vi "svx_DAQ_UpdateTriggerSection.vi"(5 "State":T1={"Channel Info Array"=[], "Timing Mode"=enum."Time", "Timing Control 1"=25600.0, "Timing Control 2"=2560.0, "Timing Control 3"=16, "Timing Indicator 1"=0.1, "Reference Visible?"=FALSE, "Reference Type"=enum."<none>", "Tachometer Channel"="", "Tach Pulses Per Rev"=1, "Tach Direction"=enum."CW", "Tach Slope"=enum."Rising", "Tach Threshold"=0.0, "Trigger Channel"="", "Trigger Level"=20.0, "Pretrigger Samples"=1, "Trigger Slope"=enum."Falling", "Trigger Hysteresis"=0.0, "Logging Visible?"=FALSE, "Enable Logging"=FALSE, "Logfile Path"=path "c:/test.tdms"} {"Timing Control 2" format="%#_6f"; "Channel Info Array"."Max" min=0.0 format="± %^#_4g"; "Channel Info Array"."Channel Type" items=["Voltage (V)"=0, "Charge (C)"=9, "-"=99, "SPL (Pa)"=3, "Force (lbf)"=6, "Force (N)"=1, "Acceleration (g) - IEPE"=2, "Acceleration (g) - Charge"=12, "Acceleration (g) - 4 wire DC Voltage"=22, "Velocity (in/s)"=7, "Velocity (mm/s)"=8, "Prox Probe (mil)"=4, "Prox Probe (mm)"=5]}, 9 "Reference Cluster":T11, 11 "error in (no error)":errorcluster) -> (6 "State Out":T1={"Channel Info Array"=[], "Timing Mode"=enum."Time", "Timing Control 1"=25600.0, "Timing Control 2"=2560.0, "Timing Control 3"=16, "Timing Indicator 1"=0.1, "Reference Visible?"=FALSE, "Reference Type"=enum."<none>", "Tachometer Channel"="", "Tach Pulses Per Rev"=1, "Tach Direction"=enum."CW", "Tach Slope"=enum."Rising", "Tach Threshold"=0.0, "Trigger Channel"="", "Trigger Level"=20.0, "Pretrigger Samples"=1, "Trigger Slope"=enum."Falling", "Trigger Hysteresis"=0.0, "Logging Visible?"=FALSE, "Enable Logging"=FALSE, "Logfile Path"=path "c:/test.tdms"} caption="State" {"Timing Control 2" format="%#_6f"; "Channel Info Array"."Max" min=0.0 format="± %^#_4g"; "Channel Info Array"."Channel Type" items=["Voltage (V)"=0, "Charge (C)"=9, "-"=99, "SPL (Pa)"=3, "Force (lbf)"=6, "Force (N)"=1, "Acceleration (g) - IEPE"=2, "Acceleration (g) - Charge"=12, "Acceleration (g) - 4 wire DC Voltage"=22, "Velocity (in/s)"=7, "Velocity (mm/s)"=8, "Prox Probe (mil)"=4, "Prox Probe (mm)"=5]}, 10 "Reference Cluster Out":T11, 15 "error out":errorcluster)   [LabVIEW 2017, in "SVX NI-DAQmx AI Configuration XControl.xctl"]
uses:
  <vilib>/addons/Sound and Vibration/svt_DAQmx/Configuration XControl/SVX NI-DAQmx AI Configuration XControl.xctl
  <vilib>/addons/Sound and Vibration/svt_DAQmx/Configuration XControl/SubVIs/svx_DAQ_State.ctl
  <vilib>/addons/Sound and Vibration/svt_DAQmx/Configuration XControl/Controls/svx_DAQ_ChannelInfo.ctl
  <vilib>/addons/Sound and Vibration/svt_DAQmx/Configuration XControl/Controls/svx_DAQ_ChannelType.ctl
  <vilib>/addons/Sound and Vibration/svt_DAQmx/Configuration XControl/Controls/svx_DAQ_Coupling.ctl
  <vilib>/addons/Sound and Vibration/svt_DAQmx/Configuration XControl/Controls/svx_DAQ_Excitation.ctl
  <vilib>/addons/Sound and Vibration/svt_DAQmx/Configuration XControl/Controls/svx_DAQ_TimingType.ctl
  <vilib>/addons/Sound and Vibration/svt_DAQmx/Configuration XControl/Controls/svx_DAQ_ReferenceType.ctl
  <vilib>/addons/Sound and Vibration/svt_DAQmx/Configuration XControl/Controls/svx_DAQ_RotationDirection.ctl
  <vilib>/addons/Sound and Vibration/svt_DAQmx/Configuration XControl/Controls/svx_DAQ_Tach_Slope.ctl
  <vilib>/addons/Sound and Vibration/svt_DAQmx/Configuration XControl/Controls/svx_DAQ_Trigger_Slope.ctl
  <vilib>/addons/Sound and Vibration/svt_DAQmx/Configuration XControl/Controls/svx_DAQ_ControlRefs.ctl
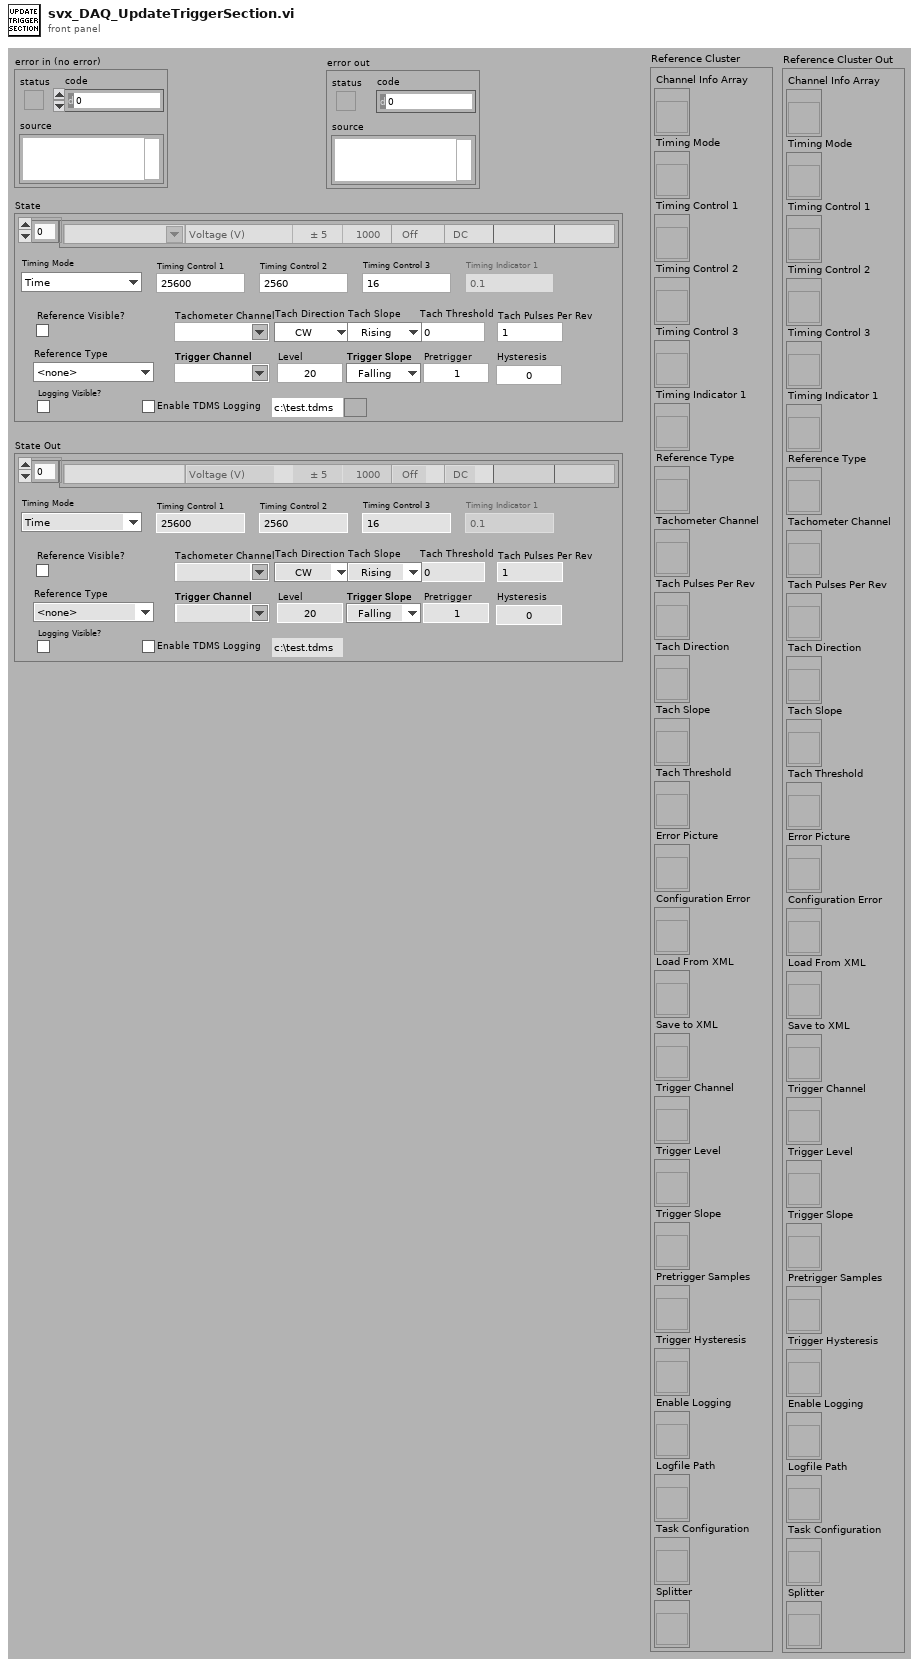
[diagram p1: front panel]
types:
  T1 = typedef "SVX NI-DAQmx AI Configuration XControl.xctl/svx_DAQ_State.ctl" = cluster{"Channel Info Array":T2[], "Timing Mode":T6, "Timing Control 1":dbl, "Timing Control 2":dbl, "Timing Control 3":i32, "Timing Indicator 1":dbl, "Reference Visible?":bool, "Reference Type":T7, "Tachometer Channel":string, "Tach Pulses Per Rev":i32, "Tach Direction":T8, "Tach Slope":T9, "Tach Threshold":dbl, "Trigger Channel":string, "Trigger Level":dbl, "Pretrigger Samples":i32, "Trigger Slope":T10, "Trigger Hysteresis":dbl, "Logging Visible?":bool, "Enable Logging":bool, "Logfile Path":path}
  T2 = typedef "SVX NI-DAQmx AI Configuration XControl.xctl/svx_DAQ_ChannelInfo.ctl" = cluster{"Initialized?":bool, "DAQmx Channel":tag, "Channel Type":T3, "Max":dbl, "Sensitivity":dbl, "Excitation":bool, "Coupling":T4, "Location":string, "Orientation":string, "excitation":T5}
  T3 = typedef "SVX NI-DAQmx AI Configuration XControl.xctl/svx_DAQ_ChannelType.ctl" = u16
  T4 = typedef "SVX NI-DAQmx AI Configuration XControl.xctl/svx_DAQ_Coupling.ctl" = enum16{"AC", "DC"}
  T5 = typedef "svx_DAQ_Excitation.ctl" = enum16{"Off", "Min", "Max"}
  T6 = typedef "SVX NI-DAQmx AI Configuration XControl.xctl/svx_DAQ_TimingType.ctl" = enum16{"Time", "Frequency", "Order"}
  T7 = typedef "SVX NI-DAQmx AI Configuration XControl.xctl/svx_DAQ_ReferenceType.ctl" = enum16{"<none>", "Analog Tachometer", "Analog SW Trigger"}
  T8 = typedef "SVX NI-DAQmx AI Configuration XControl.xctl/svx_DAQ_RotationDirection.ctl" = enum16{"CW", "CCW"}
  T9 = typedef "SVX NI-DAQmx AI Configuration XControl.xctl/svx_DAQ_Tach_Slope.ctl" = enum16{"Rising", "Falling"}
  T10 = typedef "SVX NI-DAQmx AI Configuration XControl.xctl/svx_DAQ_Trigger_Slope.ctl" = enum16{"Falling", "Rising"}
  T11 = typedef "SVX NI-DAQmx AI Configuration XControl.xctl/svx_DAQ_ControlRefs.ctl" = cluster{"Channel Info Array":refnum<vi>, "Timing Mode":refnum<vi>, "Timing Control 1":refnum<vi>, "Timing Control 2":refnum<vi>, "Timing Control 3":refnum<vi>, "Timing Indicator 1":refnum<vi>, "Reference Type":refnum<vi>, "Tachometer Channel":refnum<vi>, "Tach Pulses Per Rev":refnum<vi>, "Tach Direction":refnum<vi>, "Tach Slope":refnum<vi>, "Tach Threshold":refnum<vi>, "Error Picture":refnum<vi>, "Configuration Error":refnum<vi>, "Load From XML":refnum<vi>, "Save to XML":refnum<vi>, "Trigger Channel":refnum<vi>, "Trigger Level":refnum<vi>, "Trigger Slope":refnum<vi>, "Pretrigger Samples":refnum<vi>, "Trigger Hysteresis":refnum<vi>, "Enable Logging":refnum<vi>, "Logfile Path":refnum<vi>, "Task Configuration":refnum<vi>, "Splitter":refnum<vi>}
  T12 = enum8{"Enabled", "Disabled", "Disabled and Grayed Out"}
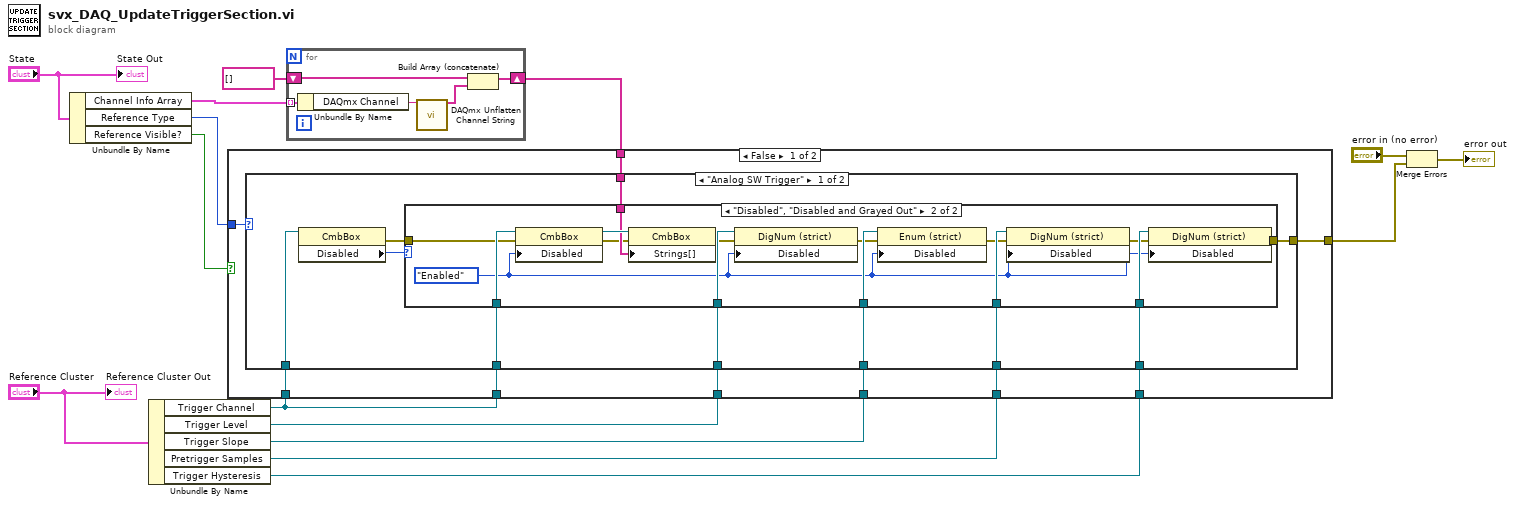
[diagram p0: block diagram]
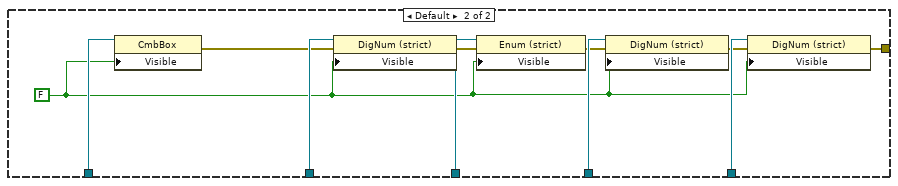
[diagram p3: hidden frame]
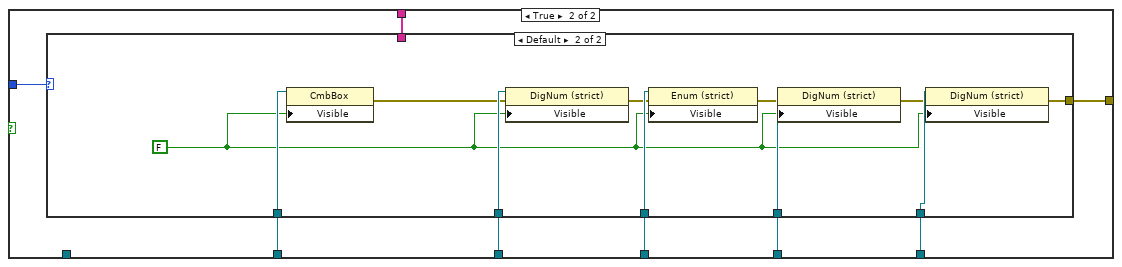
[diagram p4: hidden frame]
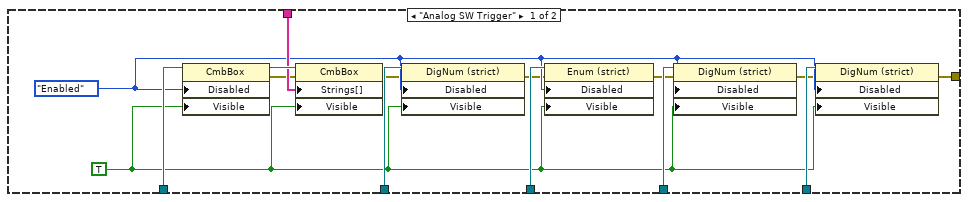
[diagram p5: hidden frame]
diagram:
  n1 = Unbundle By Name("State") -> ("Channel Info Array"=w11:T2[], "Reference Type"=w6:T7, "Reference Visible?"=w2:bool)
  n2 = Unbundle By Name("Reference Cluster") -> ("Trigger Channel"=w1:refnum<vi>, "Trigger Level"=w14:refnum<vi>, "Trigger Slope"=w15:refnum<vi>, "Pretrigger Samples"=w13:refnum<vi>, "Trigger Hysteresis"=w12:refnum<vi>)
  n3 = for {
    tunnel: w11 -> [w20] mode=indexing
    shift-right: [w17] -> w9
    shift-left: string[] [] ("Strings []") -> [w18]
    n4 = Unbundle By Name(w20) -> ("DAQmx Channel"=w19:tag)
    n5 = call <vilib>:"DAQmx Unflatten Channel String.vi"("names in"=w19) -> ("names out"=w16:string[])  [unwired: 13 in, 1 out]
    n6 = Build Array (concatenate)(w18, w16) -> (w17:string[])
  }
  n7 = case shown="False" w2 {
    tunnel: w15 -> [w24 w74]
    tunnel: w14 -> [w25 w73]
    tunnel: w13 -> [w23 w72]
    tunnel: w12 -> [w22 w71]
    tunnel: w9 -> [w27 w70]
    tunnel: [w29 w69] -> w8
    tunnel: w6 -> [w28 w68]
    tunnel: w1 -> [w26 w67]
    tunnel: w1 -> [w21 _]
    frame False {
      n8 = case shown="\"Analog SW Trigger\"" w28 {
        tunnel: w24 -> [w39 w66]
        tunnel: w25 -> [w38 w65]
        tunnel: w26 -> [w37 w64]
        tunnel: w23 -> [w36 w63]
        tunnel: w22 -> [w35 w62]
        tunnel: w27 -> [w34 _]
        tunnel: [w33 w58] -> w29
        tunnel: w21 -> [w32 _]
        frame "Analog SW Trigger" {
          n9 = property class="CmbBox"(reference=w32) -> (error out=w30:errorcluster, "Disabled"=w31:T12)  [unwired: 1 in, 1 out]
          n10 = case shown="\"Disabled\", \"Disabled and Grayed Out\"" w31 {
            tunnel: w39 -> [_ w55]
            tunnel: w38 -> [_ w54]
            tunnel: w37 -> [_ w53]
            tunnel: w36 -> [_ w52]
            tunnel: w35 -> [_ w51]
            tunnel: w34 -> [_ w49]
            tunnel: [w40 w43] -> w33
            tunnel: w30 -> [w40 w41]
            frame "Enabled", Default {
            }
            frame "Disabled", "Disabled and Grayed Out" {
              w42 = T12."Enabled" ("Disabled")
              n11 = property class="CmbBox"(reference=w53, error in=w41, "Disabled"=w42) -> (reference out=w50:refnum<vi>, error out=w48:errorcluster)
              n12 = property class="CmbBox"(reference=w50, error in=w48, "Strings[]"=w49) -> (error out=w47:errorcluster)  [unwired: 1 out]
              n13 = property class="DigNum (strict)"(reference=w54, error in=w47, "Disabled"=w42) -> (error out=w46:errorcluster)  [unwired: 1 out]
              n14 = property class="Enum (strict)"(reference=w55, error in=w46, "Disabled"=w42) -> (error out=w45:errorcluster)  [unwired: 1 out]
              n15 = property class="DigNum (strict)"(reference=w52, error in=w45, "Disabled"=w42) -> (error out=w44:errorcluster)  [unwired: 1 out]
              n16 = property class="DigNum (strict)"(reference=w51, error in=w44, "Disabled"=w42) -> (error out=w43:errorcluster)  [unwired: 1 out]
            }
          }
        }
        frame Default {
          w56 = FALSE ("Visible")
          n17 = property class="CmbBox"(reference=w64, "Visible"=w56) -> (error out=w57:errorcluster)  [unwired: 1 in, 1 out]
          n18 = property class="DigNum (strict)"(reference=w65, error in=w57, "Visible"=w56) -> (error out=w61:errorcluster)  [unwired: 1 out]
          n19 = property class="Enum (strict)"(reference=w66, error in=w61, "Visible"=w56) -> (error out=w60:errorcluster)  [unwired: 1 out]
          n20 = property class="DigNum (strict)"(reference=w63, error in=w60, "Visible"=w56) -> (error out=w59:errorcluster)  [unwired: 1 out]
          n21 = property class="DigNum (strict)"(reference=w62, error in=w59, "Visible"=w56) -> (error out=w58:errorcluster)  [unwired: 1 out]
        }
      }
    }
    frame True {
      n22 = case shown="Default" w68 {
        tunnel: w74 -> [w89 w100]
        tunnel: w73 -> [w88 w99]
        tunnel: w67 -> [w87 w98]
        tunnel: w72 -> [w86 w97]
        tunnel: w71 -> [w85 w96]
        tunnel: w70 -> [w83 _]
        tunnel: [w76 w92] -> w69
        frame "Analog SW Trigger" {
          w75 = TRUE ("Visible")
          w82 = T12."Enabled" ("Disabled")
          n23 = property class="CmbBox"(reference=w87, "Disabled"=w82, "Visible"=w75) -> (reference out=w84:refnum<vi>, error out=w81:errorcluster)  [unwired: 1 in]
          n24 = property class="CmbBox"(reference=w84, error in=w81, "Strings[]"=w83, "Visible"=w75) -> (error out=w80:errorcluster)  [unwired: 1 out]
          n25 = property class="DigNum (strict)"(reference=w88, error in=w80, "Disabled"=w82, "Visible"=w75) -> (error out=w79:errorcluster)  [unwired: 1 out]
          n26 = property class="Enum (strict)"(reference=w89, error in=w79, "Disabled"=w82, "Visible"=w75) -> (error out=w78:errorcluster)  [unwired: 1 out]
          n27 = property class="DigNum (strict)"(reference=w86, error in=w78, "Disabled"=w82, "Visible"=w75) -> (error out=w77:errorcluster)  [unwired: 1 out]
          n28 = property class="DigNum (strict)"(reference=w85, error in=w77, "Disabled"=w82, "Visible"=w75) -> (error out=w76:errorcluster)  [unwired: 1 out]
        }
        frame Default {
          w90 = FALSE ("Visible")
          n29 = property class="CmbBox"(reference=w98, "Visible"=w90) -> (error out=w91:errorcluster)  [unwired: 1 in, 1 out]
          n30 = property class="DigNum (strict)"(reference=w99, error in=w91, "Visible"=w90) -> (error out=w95:errorcluster)  [unwired: 1 out]
          n31 = property class="Enum (strict)"(reference=w100, error in=w95, "Visible"=w90) -> (error out=w94:errorcluster)  [unwired: 1 out]
          n32 = property class="DigNum (strict)"(reference=w97, error in=w94, "Visible"=w90) -> (error out=w93:errorcluster)  [unwired: 1 out]
          n33 = property class="DigNum (strict)"(reference=w96, error in=w93, "Visible"=w90) -> (error out=w92:errorcluster)  [unwired: 1 out]
        }
      }
    }
  }
  n34 = Merge Errors("error in (no error)", w8) -> (→"error out":errorcluster)
  "Reference Cluster Out" <- "Reference Cluster"
  "State Out" <- "State"
